vi "Register for Events.vi"(8 "Error In":errorcluster, 11 "Panel Actor in":refnum<class "Panel Actor.lvclass">) -> (0 "Error Out":errorcluster, 3 "Panel Actor out":refnum<class "Panel Actor.lvclass">, 5 "Pnl Actor":refnum<event-registration> caption="Panel Actor Events", 7 "Self Enqueuer":refnum<class "Message Enqueuer.lvclass">)   [LabVIEW 2019, in "Panel Actor.lvlib" / "Panel Actor.lvclass"]
doc: "Registers for the Actor Events. The self Enqueuer is returned for convenience.\n\nNote: This VI will register for events even on error in. This is to ensure your Event Handler loop will get the stop even event if an error has been generated.\n\n<B>Panel Actor In:</B> Panel Actor object\n<B>Offset:</B> Input Offset object.\n<B>Self Enqueuer:</B> Self Enqueuer object.\n<B>Panel Actor Events:</B> Event Registration refnum for panel-defined user events.\n<B>Error In:</B> Describes error conditions that occur before this node runs.\n\n<B>Panel Actor Out:</B> Panel Actor object.\n<B>Error Out:</B> Contains error information.\n----\nPlease see the following web address for additional documentation and tutorial information:\nhttp://www.mooregoodideas.com/mgi-panel-manager/\n\nAuthor: Derek Trepanier\n\nCopyright (c) 2018, Moore Good Ideas, Inc.\n\nAll rights reserved.\n\nRedistribution and use in source and binary forms, with or without modification, are permitted provided that the following conditions are met:\n\n * Redistributions of source code must retain the above copyright notice, this list of conditions and the following disclaimer.\n * Redistributions in binary form must reproduce the above copyright notice, this list of conditions and the following disclaimer in the documentation and/or other materials provided with the distribution.\n * Neither the name of Moore Good Ideas, Inc. nor the names of its contributors may be used to endorse or promote products derived from this software without specific prior written permission.\n\nTHIS SOFTWARE IS PROVIDED BY THE COPYRIGHT HOLDERS AND CONTRIBUTORS \"AS IS\" AND ANY EXPRESS OR IMPLIED WARRANTIES, INCLUDING, BUT NOT LIMITED TO, THE IMPLIED WARRANTIES OF MERCHANTABILITY AND FITNESS FOR A PARTICULAR PURPOSE ARE DISCLAIMED. IN NO EVENT SHALL THE COPYRIGHT OWNER OR CONTRIBUTORS BE LIABLE FOR ANY DIRECT, INDIRECT, INCIDENTAL, SPECIAL, EXEMPLARY, OR CONSEQUENTIAL DAMAGES (INCLUDING, BUT NOT LIMITED TO, PROCUREMENT OF SUBSTITUTE GOODS OR SERVICES; LOSS OF USE, DATA, OR PROFITS; OR BUSINESS INTERRUPTION) HOWEVER CAUSED AND ON ANY THEORY OF LIABILITY, WHETHER IN CONTRACT, STRICT LIABILITY, OR TORT (INCLUDING NEGLIGENCE OR OTHERWISE) ARISING IN ANY WAY OUT OF THE USE OF THIS SOFTWARE, EVEN IF ADVISED OF THE POSSIBILITY OF SUCH DAMAGE."
uses:
  Panel Actor.lvclass
  builds/Engine/Actor Framework.lvlibp/1abvi3w/vi.lib/ActorFramework/Actor/Actor.lvclass
  C:/Users/Public/Documents/Development/builds/Engine/Monitored Actor.lvlibp/Monitored Actor/Monitored Actor/Monitored Actor.lvclass
  C:/Users/Public/Documents/Development/builds/Engine/Actor Framework.lvlibp/1abvi3w/vi.lib/ActorFramework/Actor/Actor.lvclass
  builds/Engine/Panel.lvlibp/Panel Helper/Events.ctl
  builds/Engine/Panel.lvlibp/Panel Helper/Panel Helper.lvclass
  builds/Engine/Panel.lvlibp/Panel Helper/Panel Events.ctl
  builds/Engine/Actor Framework.lvlibp/1abvi3w/vi.lib/ActorFramework/Message Enqueuer/Message Enqueuer.lvclass
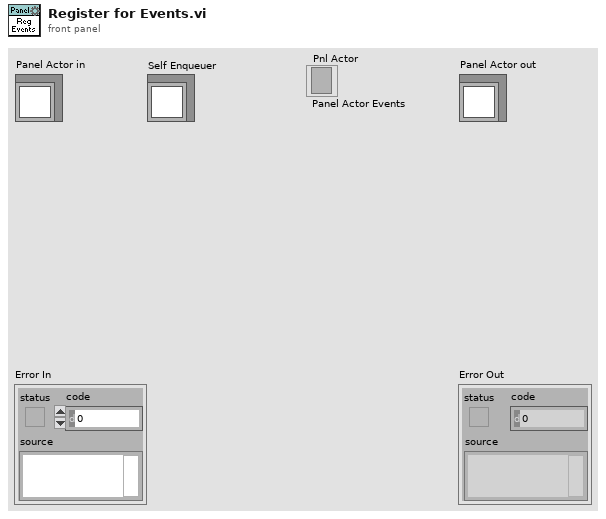
[diagram p1: front panel]
types:
  T1 = cluster{"Initialized":refnum<user-event>, "Stopped":refnum<user-event>}
  T2 = typedef "Panel.lvlibp/Panel Helper.lvclass/Panel Events.ctl" = cluster{"My Panel":refnum<user-event>, "Top Level Initialized":refnum<user-event>}
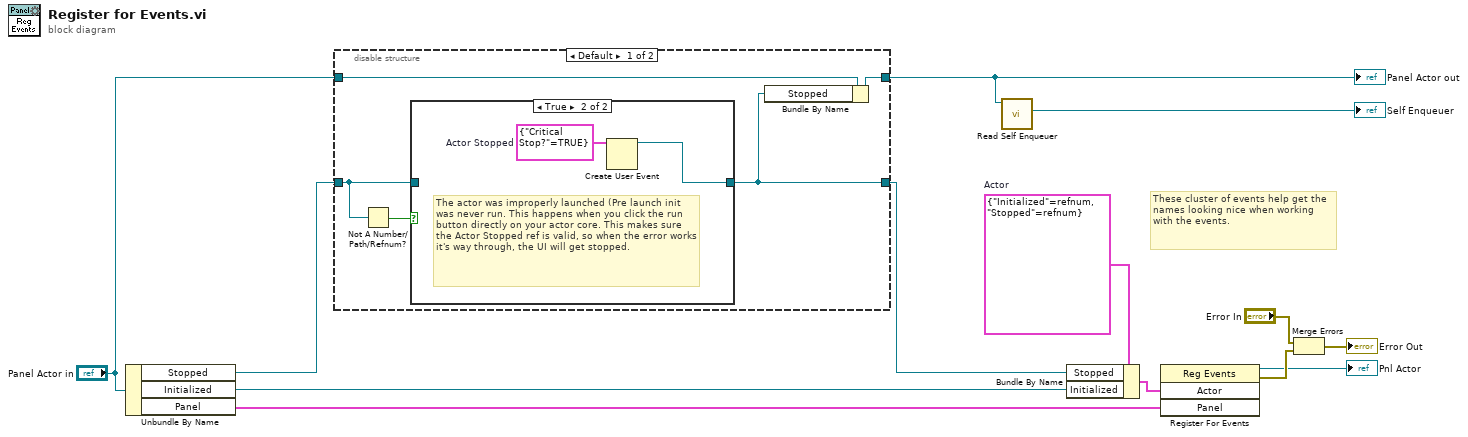
[diagram p0: block diagram]
diagram:
  w8 = T1 {"Initialized"=refnum, "Stopped"=refnum}  # Actor
  # "These cluster of events help get the names looking nice when working with the events."
  n1 = Unbundle By Name("Panel Actor in") -> ("Stopped"=w10:refnum<user-event>, "Initialized"=w5:refnum<user-event>, "Panel"=w4:T2)
  n2 = disable-structure shown="Default" {
    disable-tunnel: w10 -> [w17 w23]
    disable-tunnel: [w14 w23] -> w6
    disable-tunnel: [w15 w22] -> w2
    disable-tunnel: "Panel Actor in" -> [w16 w22]
    frame condition #0 (active) {
      n3 = Not A Number/Path/Refnum?(number/path/refnum=w17) -> (NaN/Path/Refnum?=w18:bool)
      n4 = case shown="True" w18 {
        tunnel: w17 -> [w19 _]
        tunnel: [w19 w20] -> w14
        frame False {
        }
        frame True {
          w21 = cluster{"Critical Stop?":bool} {"Critical Stop?"=TRUE}  # Actor Stopped
          # "The actor was improperly launched (Pre launch init was never run. This happens when you click the run button directly on your actor core. This makes sure the Actor Stopped ref is valid, so when the error works it's way through, the UI will get stopped."
          n5 = Create User Event(user event datatype=w21) -> (user event=w20:refnum<user-event>)  [unwired: 1 in, 1 out]
        }
      }
      n6 = Bundle By Name(cluster=w16, "Stopped"=w14) -> (w15:refnum<class "Panel Actor.lvclass">)
    }
    frame condition #1 {
      # "The actor can only get improperly launched in the dev enviroment."
    }
  }
  "Panel Actor out" <- w2
  n7 = call "Read Self Enqueuer.vi"("Actor"=w2) -> ("Self Enqueuer"=→"Self Enqueuer":refnum<class "Message Enqueuer.lvclass">)  [unwired: 10 in]
  n8 = Bundle By Name(cluster=w8, "Stopped"=w6, "Initialized"=w5) -> (w7:T1)
  n9 = register-events(w7, w4) -> (reference out=→"Pnl Actor":refnum<event-registration>, error out=w11:errorcluster)  [unwired: 2 in]
  n10 = Merge Errors("Error In", w11) -> (→"Error Out":errorcluster)
